vi "DPO.vi"(0 "System no.":i32=1 min=1 max=4 step=1, 2 "DPO axes":string[](array[string]), 3 "All axes?":bool, 4 "Axis identifier?":bool=TRUE, 5 "error in":errorcluster) -> (19 "error out":errorcluster)   [LabVIEW 2020]
doc: "DDL processing parameter correction for specified axis. Calculates internal DDL processing parameters. DPO is required when servo parameters have changed for an axis.\n\nE-710: If All axes = TRUE, then Axis identifier must be TRUE. Command is available in command level 1 only (see CCL.vi and CCL?.vi)\nE-712: If All axes? = TRUE, then Axis identifier? can be FALSE\nE-725, E-727: If All axes? = TRUE, then Axis identifier? can be FALSE\nE-753, E-754: If All axes = TRUE, then Axis identifier? can be FALSE."
panel:
  # "DDL processing parameter correction for \nspecified axis."
  # "If all axes: use"
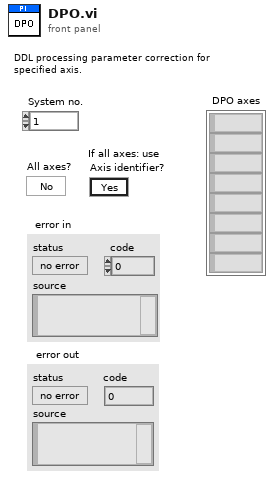
[diagram p1: front panel]
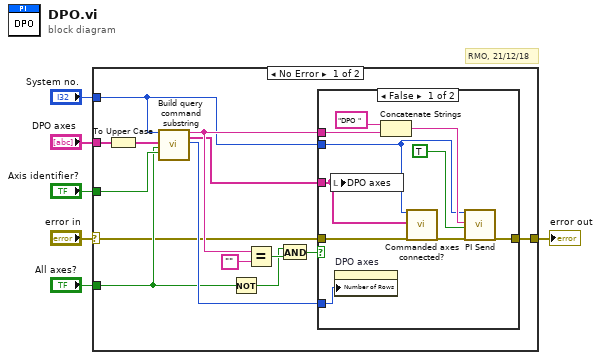
[diagram p0: block diagram]
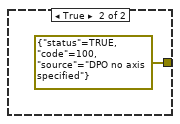
[diagram p2: hidden frame]
diagram:
  # "RMO, 21/12/18"
  n1 = case shown="No Error" "error in" {
    selector: "error in" -> [w9 w32]
    tunnel: "DPO axes" -> [w20 _]
    tunnel: "Axis identifier?" -> [w17 _]
    tunnel: "System no." -> [w15 _]
    tunnel: "All axes?" -> [w11 _]
    tunnel: [w8 w32] -> w2
    frame No Error {
      n2 = To Upper Case(1:w20) -> (0:w18:string[])
      n3 = call "Build query command substring.vi"("System no."=w15, "Axes to query in"=w18, "Query\nAll axes?"=w11, "For all axes: use\nAxis identifier?"=w17) -> ("Command substring"=w16:string, "Axes to query out"=w14:string[], "Number of rows"=w13:u32)  [unwired: 2 in, 11 out]
      n4 = Not(x=w11) -> (.not. x?=w10:bool)
      n5 = Equal?(x=w16, y="" ("x")) -> (x = y?=w12:bool)
      n6 = And(x=w10, y=w12) -> (x .and. y?=w7:bool)
      n7 = case shown="False" w7 {
        tunnel: w16 -> [w27 _]
        tunnel: w15 -> [w26 _]
        tunnel: w14 -> [w25 _]
        tunnel: w13 -> [w23 _]
        tunnel: w9 -> [w22 _]
        tunnel: [w21 errorcluster {"status"=TRUE, "code"=100, "source"="DPO no axis specified"} ("error out")] -> w8
        frame False {
          n8 = local write "DPO axes"(w25) -> ()
          n9 = property on="DPO axes" class="Arr (strict)"("Number of Rows"=w23) -> ()  [unwired: 2 in, 2 out]
          n10 = Concatenate Strings("DPO ", w27) -> (w28:string)
          n11 = call "Commanded axes connected?.vi"("System no."=w26, "Commanded axes"=w25, "error in"=w22) -> ("error out"=w24:errorcluster)  [unwired: 1 in, 15 out]
          n12 = call "PI Send.vi"("System no."=w26, "String to send"=w28, "Attach termination char.?"=TRUE ("Attach Linefeed?"), "error in"=w24) -> ("error out"=w21:errorcluster)  [unwired: 2 in, 13 out]
        }
        frame True {
        }
      }
    }
    frame Error {
    }
  }
  "error out" <- w2
